vi "niFPGALMRsmplLMInSCTL.vi"(0 "input data":fxp<+/-,16,1>, 1 "reset":bool, 9 "input valid":bool, 12 "ready for output":bool) -> (3 "channel index":u8, 4 "output data":fxp<+/-,18,1> format="%.18g", 10 "output valid":bool, 14 "ready for input":bool)   [LabVIEW 2017]
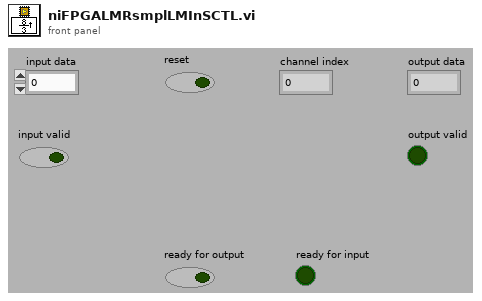
[diagram p1: front panel]
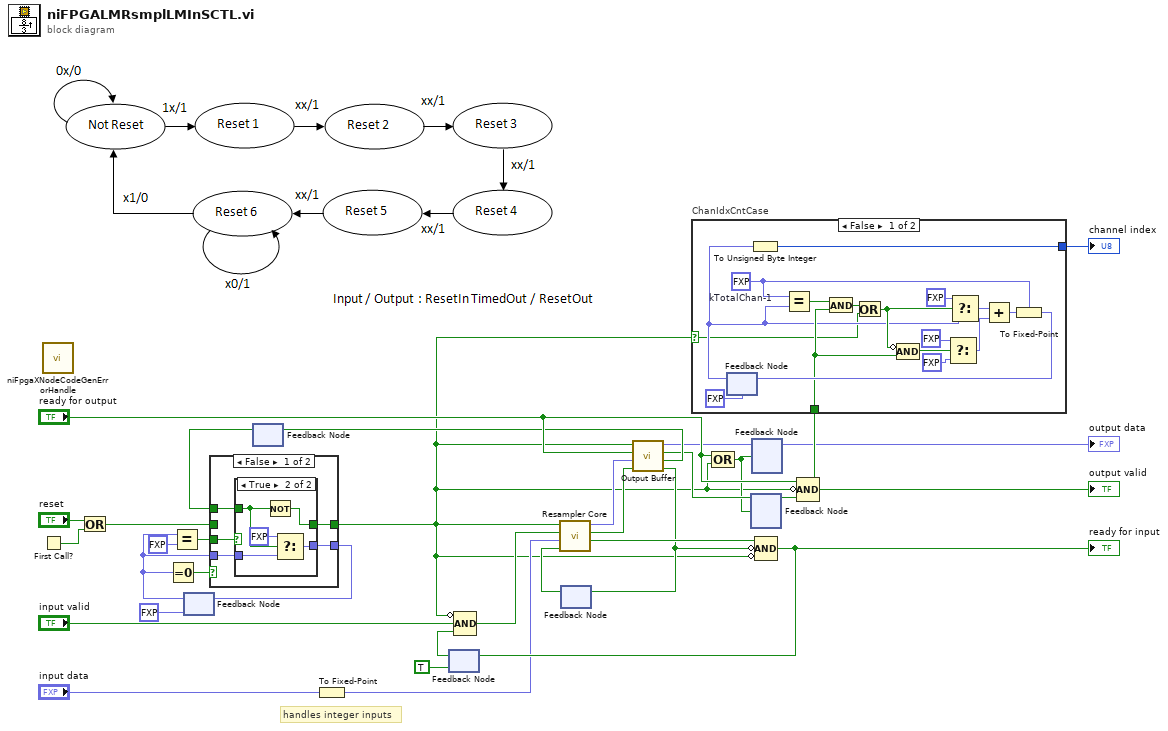
[diagram p0: block diagram]
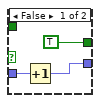
[diagram p2: hidden frame]
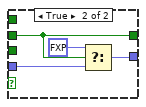
[diagram p3: hidden frame]
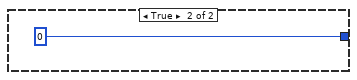
[diagram p4: hidden frame]
diagram:
  # "handles integer inputs"
  n1 = First Call?() -> (First Call?: T/F=w31:bool)
  n2 = call <vilib>:"niFpgaXNodeCodeGenErrorHandle.vi"() -> ()  [unwired: 1 in]
  n3 = Or(x="reset", y=w31) -> (x .or. y?=w2:bool)
  n4 = feedback #1(fxp<+,3,3> 0.0) -> (w7:fxp<+,3,3>)
  n5 = Equal To 0?(x=w7) -> (x = 0?=w8:bool)
  n6 = Equal?(x=w7, y=fxp<+,3,3> 6.0) -> (x = y?=w5:bool)
  n7 = feedback #2() -> (w3:bool)  [unwired: 1 in]
  n8 = case shown="False" w8 {
    tunnel: w2 -> [_ w48]
    tunnel: [w34 w49] -> w4
    tunnel: [w36 w48] -> w1
    tunnel: w7 -> [w35 w47]
    tunnel: w5 -> [w37 _]
    tunnel: w3 -> [w33 _]
    frame False {
      n9 = case shown="True" w37 {
        tunnel: [TRUE w45] -> w36
        tunnel: w35 -> [w39 w41]
        tunnel: [w38 w44] -> w34
        tunnel: w33 -> [_ w43]
        frame False {
          n10 = Increment(x=w39) -> (x+1=w38:fxp<+,3,3>)
        }
        frame True {
          n11 = Not(x=w43) -> (.not. x?=w45:bool)
          n12 = Select(t=fxp<+,3,3> 0.0, s=w43, f=w41) -> (s? t:f=w44:fxp<+,3,3>)
        }
      }
    }
    frame True {
      n13 = Select(t=fxp<+,3,3> 1.0, s=w48, f=w47) -> (s? t:f=w49:fxp<+,3,3>)
    }
  }
  n14 = feedback-in #1(w4) -> ()
  n15 = To Fixed-Point(number="input data") -> (fixed-point=w10:fxp<+/-,16,1>)  [unwired: 1 in]
  n16 = feedback #3(TRUE) -> (w25:bool)
  n17 = Compound Arithmetic op=AND(invert w1, "input valid", w25) -> (w30:bool)
  n18 = feedback #4() -> (w26:bool)  [unwired: 1 out]
  n19 = call "Resampler Core"("FIFOIsFull"=w26, "datain"=w10, "dataRDYIn"=w30, "reset"=w1) -> ("idle"=w22:bool, "dataRDYOut"=w28:bool, "y"=w27:fxp<+/-,18,1>)  [unwired: 5 in]
  n20 = call "Output Buffer"("wrEn"=w28, "wrVal"=w27, "ready for output"="ready for output", "reset"=w1) -> ("wrTimedOut?"=w20:bool, "rdTimedOut?"=w17:bool, "outputValid"=w14:bool, "outputData"=w16:fxp<+/-,18,1>)  [unwired: 4 in]
  n21 = feedback-in #2(w17) -> ()
  n22 = feedback-in #4(w20) -> ()
  n23 = Compound Arithmetic op=OR("ready for output", w1) -> (w13:bool)
  n24 = feedback #5() -> (w12:bool)  [unwired: 1 in]
  n25 = feedback-in #5(w14, w13) -> ()
  n26 = feedback #6() -> (→"output data":fxp<+/-,18,1>)  [unwired: 1 in]
  n27 = feedback-in #6(w16, w13) -> ()
  n28 = Compound Arithmetic op=AND(w22, invert w20, invert w1) -> (w29:bool)
  "ready for input" <- w29
  n29 = feedback-in #3(w29) -> ()
  n30 = Compound Arithmetic op=AND("ready for output", invert w1, w12) -> (w19:bool)
  "output valid" <- w19
  n31 = case "ChanIdxCntCase" shown="False" w1 {
    selector: w1 -> [w51 _]
    tunnel: w19 -> [w53 _]
    tunnel: [w66 u8 0] -> w18
    frame False {
      w54 = fxp<+,1,1> 0.0  # kTotalChan-1
      n32 = feedback #7(fxp<+,1,1> 0.0) -> (w52:fxp<+,1,1>)
      n33 = To Unsigned Byte Integer(number=w52) -> (unsigned 8bit integer=w66:u8)
      n34 = Equal?(x=w54, y=w52) -> (x = y?=w65:bool)
      n35 = And(x=w65, y=w53) -> (x .and. y?=w64:bool)
      n36 = Or(x=w64, y=w51) -> (x .or. y?=w63:bool)
      n37 = Compound Arithmetic op=AND(invert w63, w53) -> (w60:bool)
      n38 = Select(t=fxp<+,1,1> 1.0 ("y"), s=w60, f=fxp<+,1,1> 0.0) -> (s? t:f=w57:fxp<+,1,1>)
      n39 = Select(t=fxp<+,1,1> 0.0 ("y"), s=w63, f=w52) -> (s? t:f=w61:fxp<+,1,1>)
      n40 = Add(x=w61, y=w57) -> (x+y=w56:fxp<+,2,2>)
      n41 = To Fixed-Point(fixed-point type=w54, number=w56) -> (fixed-point=w55:fxp<+,1,1>)
      n42 = feedback-in #7(w55) -> ()
    }
    frame True {
    }
  }
  "channel index" <- w18
